vi "215.Close (SubVI).vi"(8 "error in (no error)":errorcluster, 11 "VISA resource name":refnum<visa-resource-name>="COM7") -> (0 "error out":errorcluster, 1 "Motor string":string, 2 "Position string":string)   [LabVIEW 2020]
panel:
  out "Connected":bool
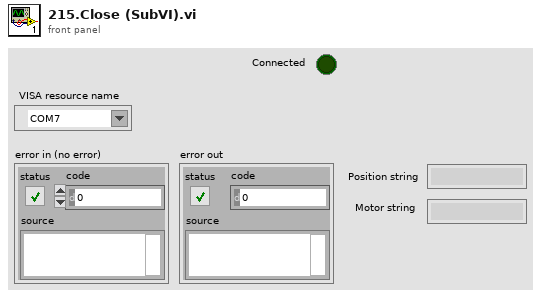
[diagram p1: front panel]
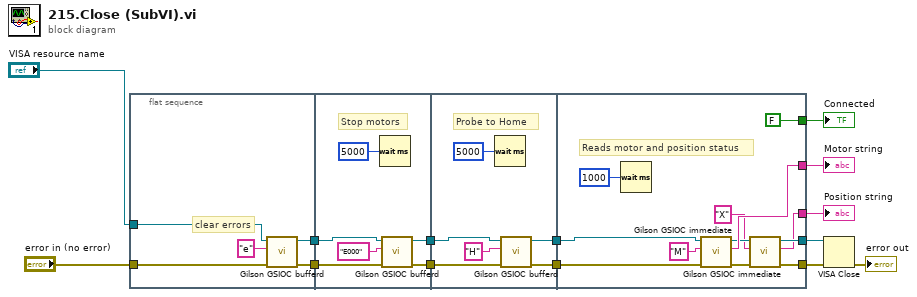
[diagram p0: block diagram]
diagram:
  n1 = flat-sequence {
    tunnel: "error in (no error)" -> [w18]
    tunnel: "VISA resource name" -> [w16]
    tunnel: [w17] -> w13
    tunnel: [w15] -> w14
    tunnel: [w25] -> w12
    tunnel: [w24] -> w11
    tunnel: w14 -> [w21]
    tunnel: w13 -> [w22]
    tunnel: w12 -> [w29]
    tunnel: w11 -> [w28]
    tunnel: [w30] -> w4
    tunnel: [w27] -> w3
    tunnel: [w34] -> w8
    tunnel: [w43] -> w6
    tunnel: [FALSE] -> w5
    tunnel: w4 -> [w39]
    tunnel: w3 -> [w38]
    tunnel: [w36] -> w2
    tunnel: [w32] -> w1
    frame #0 {
      # "clear errors"
      n2 = call <instrlib>:"Gilson GSIOC bufferd.vi"("error in (no error)"=w18, "Bufferd command"="e", "VISA resource name"=w16) -> ("error out"=w17:errorcluster, "VISA resource name out"=w15:refnum<visa-resource-name>)  [unwired: 6 in, 1 out]
    }
    frame #1 {
      # "Stop motors"
      n3 = Wait (ms)(milliseconds to wait=u32 5000) -> ()  [unwired: 1 out]
      n4 = call <instrlib>:"Gilson GSIOC bufferd.vi"("error in (no error)"=w22, "Bufferd command"="E000", "VISA resource name"=w21) -> ("error out"=w24:errorcluster, "VISA resource name out"=w25:refnum<visa-resource-name>)  [unwired: 6 in, 1 out]
    }
    frame #2 {
      # "Probe to Home"
      n5 = Wait (ms)(milliseconds to wait=u32 5000) -> ()  [unwired: 1 out]
      n6 = call <instrlib>:"Gilson GSIOC bufferd.vi"("error in (no error)"=w28, "Bufferd command"="H", "VISA resource name"=w29) -> ("error out"=w27:errorcluster, "VISA resource name out"=w30:refnum<visa-resource-name>)  [unwired: 6 in, 1 out]
    }
    frame #3 {
      # "Reads motor and position status"
      n7 = Wait (ms)(milliseconds to wait=u32 1000) -> ()  [unwired: 1 out]
      n8 = call <instrlib>:"Gilson GSIOC immediate.vi"("error in (no error)"=w38, "Immediate command"="M", "VISA resource name"=w39) -> ("error out"=w35:errorcluster, "Receive string"=w43:string, "VISA resource name"=w37:refnum<visa-resource-name>)  [unwired: 6 in]
      n9 = call <instrlib>:"Gilson GSIOC immediate.vi"("error in (no error)"=w35, "Immediate command"="X", "VISA resource name"=w37) -> ("error out"=w34:errorcluster, "Receive string"=w32:string, "VISA resource name"=w36:refnum<visa-resource-name>)  [unwired: 6 in]
    }
  }
  n10 = VISA Close(VISA resource name=w2, error in (no error)=w8) -> (error out=→"error out":errorcluster)
  "Connected" <- w5
  "Motor string" <- w6
  "Position string" <- w1
